vi "Check Config.vi"() -> ()   [LabVIEW 2022 SP3]
uses:
  Router/System Config.ctl
  Router/Mux Config.ctl
  Mux Config.ctl
  Router/Mux Links.ctl
  Web/Action.ctl
  Web/Web.lvlib
  Mux.lvclass
  Router/Router.lvclass
panel:
  out "error out":errorcluster
  out "System Config":T1
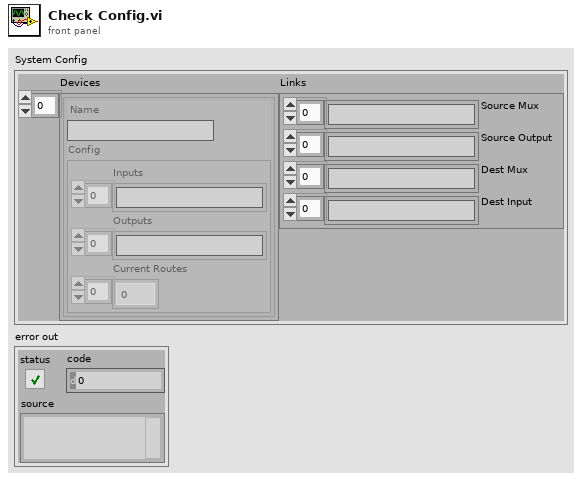
[diagram p1: front panel]
types:
  T1 = typedef "Router.lvclass/System Config.ctl" = cluster{"Devices":T2[], "Links":T4}
  T2 = typedef "Router.lvclass/Mux Config.ctl" = cluster{"Name":string, "Config":T3}
  T3 = typedef "Mux.lvclass/Mux Config.ctl" = cluster{"Inputs":string[], "Outputs":string[], "Current Routes":i32[]}
  T4 = typedef "Router.lvclass/Mux Links.ctl" = cluster{"Source Mux":string[], "Source Output":string[], "Dest Mux":string[], "Dest Input":string[]}
  T5 = typedef "Web.lvlib/Action.ctl" = enum16{"Set Router", "Apply Route", "Get Config", "Cleanup"}
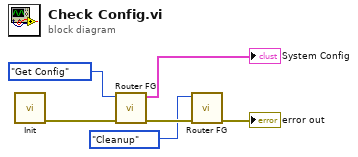
[diagram p0: block diagram]
diagram:
  n1 = call "Init.vi"() -> ("error out"=w6:errorcluster)  [unwired: 11 in]
  n2 = call "Router FG.vi"("error in (no error)"=w6, "Action"=Action."Get Config") -> ("error out"=w3:errorcluster, "System Config"=→"System Config":T1)  [unwired: 8 in]
  n3 = call "Router FG.vi"("error in (no error)"=w3, "Action"=Action."Cleanup") -> ("error out"=→"error out":errorcluster)  [unwired: 8 in, 1 out]
